vi "dvp Vi Get Quick Roi Sel.vi"(10 "pQuickRoiSel":u32, 11 "handle":u32) -> (2 "pQuickRoiSel out":u32, 3 "function return":u32(ring))   [LabVIEW 2018, in "LabViewDVPCamera.lvlib"]
doc: "LabviewDvp2Api dvpStatus dvpViGetQuickRoiSel(dvpHandle handle, dvpUint32 *pQuickRoiSel);"
uses:
  LabViewDVPCamera.lvlib
  LabViewDVPCamera/LabViewDVPCamera.dll
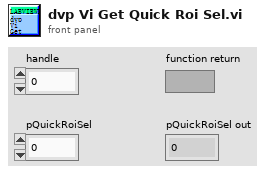
[diagram p1: front panel]
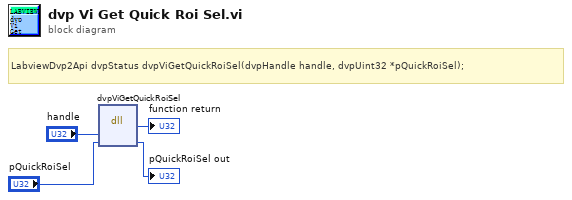
[diagram p0: block diagram]
diagram:
  # "LabviewDvp2Api dvpStatus dvpViGetQuickRoiSel(dvpHandle handle, dvpUint32 *pQuickRoiSel);"
  n1 = dll-call lib="C:/Program Files (x86)/DVP2 Labview cn 64/Sample/LabViewDVPCamera/LabViewDVPCamera.*" fn="dvpViGetQuickRoiSel"("handle"="handle", "pQuickRoiSel"="pQuickRoiSel") -> (→"function return":u32, "pQuickRoiSel"=→"pQuickRoiSel out":u32)  [unwired: 4 in, 2 out]
